vi "Select_Strings.vi"(5 "Available Ch names":string[](array[string]), 6 "Message":string, 7 "Selector mode":T1(ring), 8 "Desired Ch names (in)":string[](array[string])) -> (0 "Ch Indicies Choosen":i32[](array[numeric]), 1 "Cancel":bool, 2 "Selected Channel Names":string[](array[string]))   [LabVIEW 2010]
panel:
  in  "Cancel 1":bool
  in  "OK":bool
  in  "Search String":string
  in  "Selector":i32[](listbox)
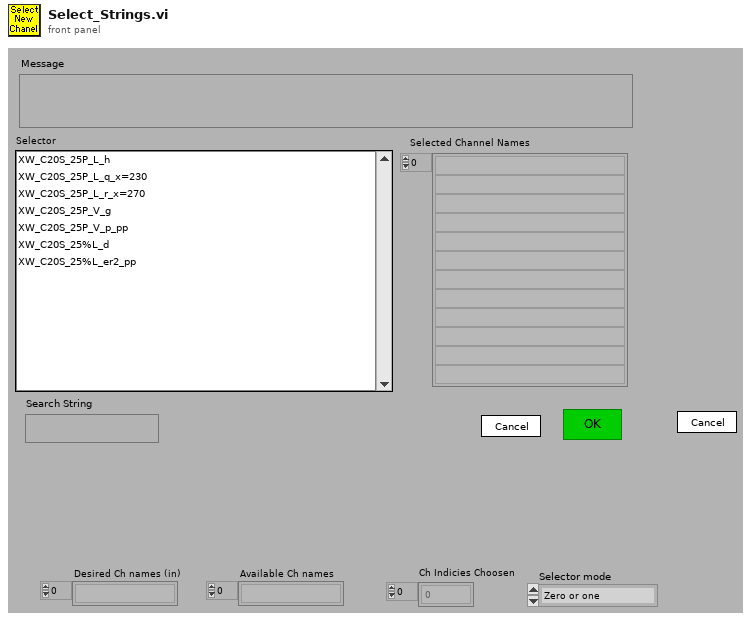
[diagram p1: front panel]
types:
  T1 = enum16{"Zero or one", "One", "Zero or more", "One or more"}
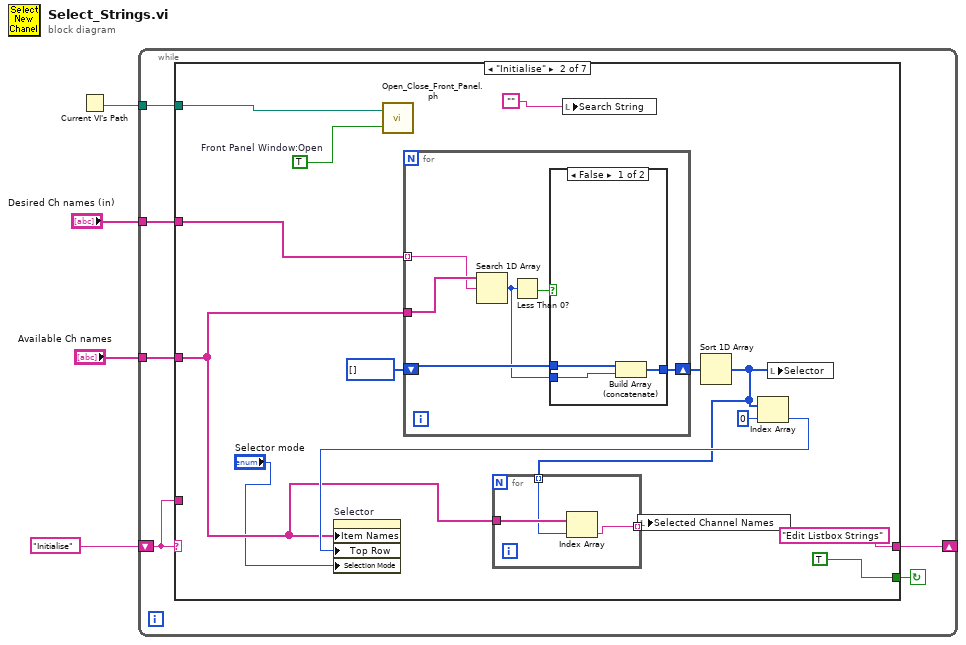
[diagram p0: block diagram]
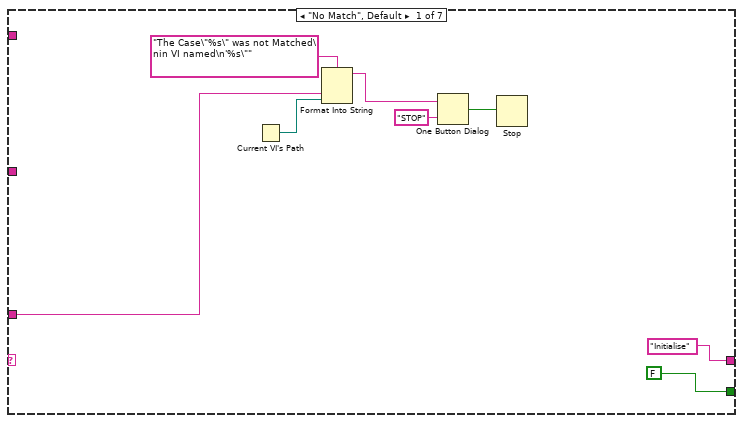
[diagram p2: hidden frame]
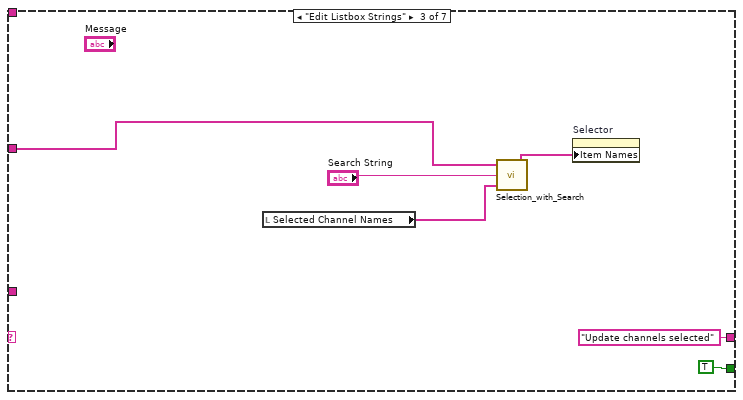
[diagram p4: hidden frame]
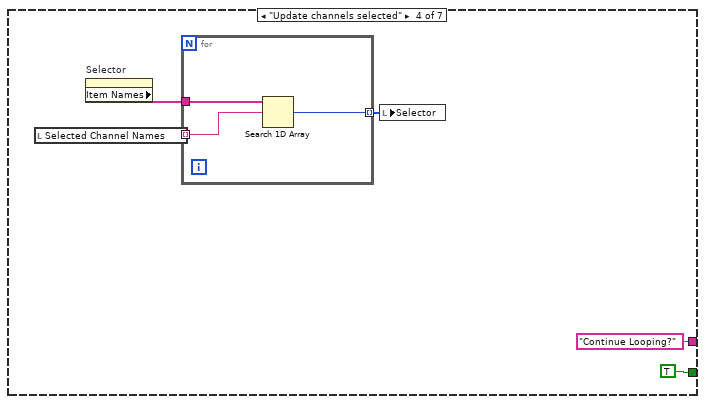
[diagram p5: hidden frame]
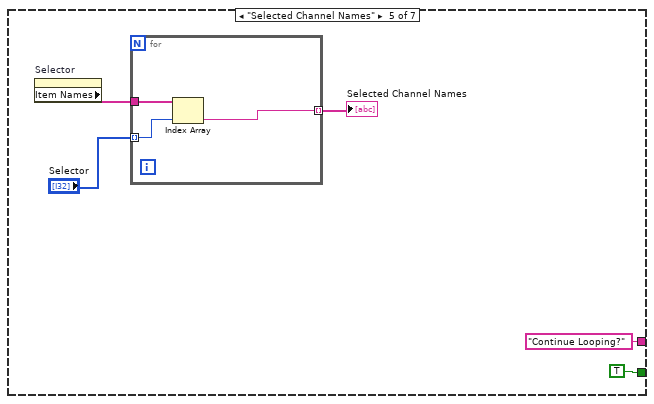
[diagram p6: hidden frame]
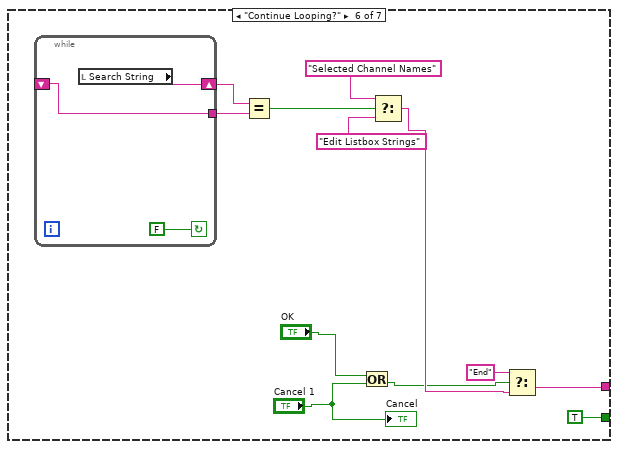
[diagram p7: hidden frame]
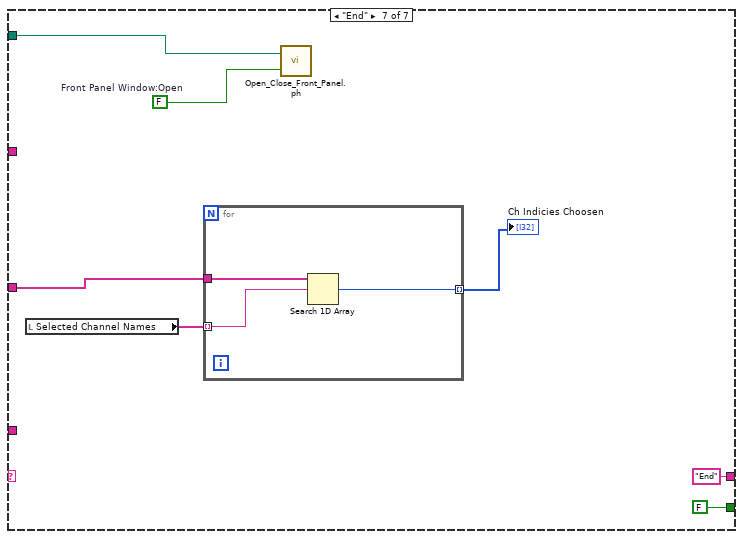
[diagram p8: hidden frame]
diagram:
  n1 = Current VI's Path() -> (path=w1:path)
  n2 = while {
    shift-left: "Initialise" -> [w8]
    shift-right: [w9] -> _
    tunnel: "Desired Ch names (in)" -> [w7]
    tunnel: "Available Ch names" -> [w6]
    tunnel: w1 -> [w5]
    stop <- w10 continue-if-true
    n3 = case shown="\"Initialise\"" w8 {
      tunnel: [FALSE TRUE TRUE TRUE TRUE TRUE FALSE] -> w10
      tunnel: ["Initialise" "Edit Listbox Strings" "Update channels selected" "Continue Looping?" "Continue Looping?" w73 "End" ("t")] -> w9
      tunnel: w8 -> [w13 _ _ _ _ _ _]
      tunnel: w7 -> [_ w27 _ _ _ _ _]
      tunnel: w6 -> [_ w25 w46 _ _ _ w87]
      tunnel: w5 -> [_ w21 _ _ _ _ w84]
      frame "No Match", Default {
        n4 = Current VI's Path() -> (path=w12:path)
        n5 = Format Into String(format string="The Case\"%s\" was not Matched\nin VI named\n'%s\"" ("Format String"), w13, w12) -> (resulting string=w16:string)  [unwired: 2 in, 1 out]
        n6 = One Button Dialog(message=w16, button name ("OK")="STOP") -> (true=w14:bool)
        n7 = Stop(stop? (T)=w14) -> ()
      }
      frame "Initialise" {
        w20 = TRUE  # Front Panel Window:Open
        n8 = call "Open_Close_Front_Panel.ph.vi"("Front Panel Window:Open"=w20, "VI path"=w21) -> ()  [unwired: 2 out]
        n9 = for {
          tunnel: w25 -> [w41]
          tunnel: w27 -> [w37] mode=indexing
          shift-right: [w38] -> w29
          shift-left: i32[] [] -> [w39]
          n10 = Search 1D Array(1D array=w41, element=w37) -> (index of element=w36:i32)  [unwired: 1 out]
          n11 = Less Than 0?(x=w36) -> (x < 0?=w40:bool)
          n12 = case shown="False" w40 {
            tunnel: w36 -> [w44 _]
            tunnel: w39 -> [w43 w45]
            tunnel: [w42 w45] -> w38
            frame False {
              n13 = Build Array (concatenate)(w43, w44) -> (w42:i32[])
            }
            frame True {
            }
          }
        }
        n14 = local write "Search String"("") -> ()
        n15 = Sort 1D Array(array=w29) -> (sorted array=w24:i32[])
        n16 = for {
          tunnel: w25 -> [w35]
          tunnel: w24 -> [w34] mode=indexing
          tunnel: [w33] -> w23 mode=indexing
          n17 = Index Array(array=w35, index=w34) -> (element=w33:string)
        }
        n18 = local write "Selected Channel Names"(w23) -> ()
        n19 = Index Array(array=w24, index=0) -> (element=w26:i32)
        n20 = property on="Selector" class="LstBox (strict)"("Item Names"=w25, "Top Row"=w26, "Selection Mode"="Selector mode") -> ()  [unwired: 2 in, 2 out]
        n21 = local write "Selector"(w24) -> ()
      }
      frame "Edit Listbox Strings" {
        n22 = local read "Selected Channel Names"() -> (w47:string[])
        n23 = call "Selection_with_Search.vi"("Selected Channel Names"=w47, "Search String"="Search String", "All Channel Names"=w46) -> ("Item Names"=w48:string[])
        n24 = property on="Selector" class="LstBox (strict)"("Item Names"=w48) -> ()  [unwired: 2 in, 2 out]
      }
      frame "Update channels selected" {
        n25 = local read "Selected Channel Names"() -> (w53:string[])
        n26 = property on="Selector" class="LstBox (strict)"() -> ("Item Names"=w54:string[])  [unwired: 2 in, 2 out]
        n27 = for {
          tunnel: w54 -> [w59]
          tunnel: w53 -> [w58] mode=indexing
          tunnel: [w57] -> w52 mode=indexing
          n28 = Search 1D Array(1D array=w59, element=w58) -> (index of element=w57:i32)  [unwired: 1 out]
        }
        n29 = local write "Selector"(w52) -> ()
      }
      frame "Selected Channel Names" {
        n30 = property on="Selector" class="LstBox (strict)"() -> ("Item Names"=w62:string[])  [unwired: 2 in, 2 out]
        n31 = for {
          tunnel: w62 -> [w67]
          tunnel: "Selector" -> [w66] mode=indexing
          tunnel: [w65] -> w60 mode=indexing
          n32 = Index Array(array=w67, index=w66) -> (element=w65:string)
        }
        "Selected Channel Names" <- w60
      }
      frame "Continue Looping?" {
        n33 = while {
          tunnel: [w81] -> w79
          shift-left: _ -> [w81]
          shift-right: [w82] -> w78
          stop <- FALSE continue-if-true
          n34 = local read "Search String"() -> (w82:string)
        }
        n35 = Equal?(x=w78, y=w79) -> (x = y?=w77:bool)
        n36 = Or(x="OK", y="Cancel 1") -> (x .or. y?=w69:bool)
        n37 = Select(t="Selected Channel Names", s=w77, f="Edit Listbox Strings") -> (s? t:f=w72:string)
        n38 = Select(t="End", s=w69, f=w72) -> (s? t:f=w73:string)
        "Cancel" <- "Cancel 1"
      }
      frame "End" {
        w83 = FALSE  # Front Panel Window:Open
        n39 = local read "Selected Channel Names"() -> (w86:string[])
        n40 = for {
          tunnel: w87 -> [w92]
          tunnel: w86 -> [w91] mode=indexing
          tunnel: [w90] -> w85 mode=indexing
          n41 = Search 1D Array(1D array=w92, element=w91) -> (index of element=w90:i32)  [unwired: 1 out]
        }
        "Ch Indicies Choosen" <- w85
        n42 = call "Open_Close_Front_Panel.ph.vi"("Front Panel Window:Open"=w83, "VI path"=w84) -> ()  [unwired: 2 out]
      }
    }
  }
